vi "HaltDev.vi"(0 "输入簇":T1) -> ()   [LabVIEW 2012]
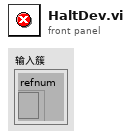
[diagram p1: front panel]
types:
  T1 = cluster{"refnum":refnum<file>, "refnum":refnum<file>, "refnum":refnum<file>, "refnum":refnum<file>, "refnum":refnum<file>, "SavePath":path, "SAVE?":bool, "connection ID":refnum<k5>}
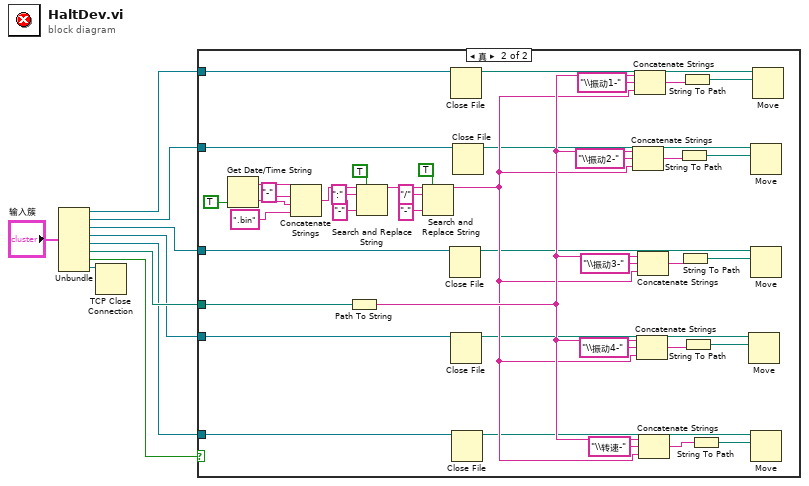
[diagram p0: block diagram]
diagram:
  n1 = Unbundle("输入簇") -> ("refnum"=w6:refnum<file>, "refnum"=w5:refnum<file>, "refnum"=w4:refnum<file>, "refnum"=w3:refnum<file>, "refnum"=w2:refnum<file>, "SavePath"=w7:path, "SAVE?"=w1:bool, "connection ID"=w8:refnum<k5>)
  n2 = TCP Close Connection(connection ID=w8) -> ()  [unwired: 2 in, 2 out]
  n3 = case shown="真" w1 {
    tunnel: w7 -> [_ w20]
    tunnel: w6 -> [_ w19]
    tunnel: w5 -> [_ w17]
    tunnel: w4 -> [_ w14]
    tunnel: w3 -> [_ w13]
    tunnel: w2 -> [_ w10]
    frame False {
    }
    frame True {
      n4 = Get Date/Time String(want seconds? (F)=TRUE ("需要秒？(F)")) -> (date string=w38:string, time string=w35:string)  [unwired: 2 in]
      n5 = Concatenate Strings(w38, "-" ("字符串"), w35, ".bin" ("字符串")) -> (w34:string)
      n6 = Path To String(path=w20) -> (string=w45:string)
      n7 = Search and Replace String(replace all?=TRUE ("替换全部？(F)"), input string=w34, search string=":" ("搜索字符串"), replace string="-" ("替换字符串(\"\")")) -> (result string=w27:string)  [unwired: 4 in, 3 out]
      n8 = Search and Replace String(replace all?=TRUE ("替换全部？(F)"), input string=w27, search string="/" ("搜索字符串"), replace string="-" ("替换字符串(\"\")")) -> (result string=w26:string)  [unwired: 4 in, 3 out]
      n9 = Close File(refnum=w14) -> (path=w15:path)  [unwired: 1 in, 1 out]
      n10 = Close File(refnum=w19) -> (path=w18:path)  [unwired: 1 in, 1 out]
      n11 = Close File(refnum=w13) -> (path=w12:path)  [unwired: 1 in, 1 out]
      n12 = Close File(refnum=w10) -> (path=w11:path)  [unwired: 1 in, 1 out]
      n13 = Close File(refnum=w17) -> (path=w16:path)  [unwired: 1 in, 1 out]
      n14 = Concatenate Strings(w45, "\\振动2-" ("字符串"), w26) -> (w47:string)
      n15 = Concatenate Strings(w45, "\\振动1-" ("字符串"), w26) -> (w46:string)
      n16 = Concatenate Strings(w45, "\\振动4-" ("字符串"), w26) -> (w49:string)
      n17 = Concatenate Strings(w45, "\\振动3-" ("字符串"), w26) -> (w48:string)
      n18 = Concatenate Strings(w45, "\\转速-" ("字符串"), w26) -> (w50:string)
      n19 = String To Path(string=w47) -> (path=w24:path)
      n20 = String To Path(string=w48) -> (path=w23:path)
      n21 = String To Path(string=w46) -> (path=w25:path)
      n22 = String To Path(string=w49) -> (path=w22:path)
      n23 = String To Path(string=w50) -> (path=w21:path)
      n24 = Move(source path=w12, 10:w22) -> ()  [unwired: 3 in, 3 out]
      n25 = Move(source path=w16, 10:w24) -> ()  [unwired: 3 in, 3 out]
      n26 = Move(source path=w15, 10:w23) -> ()  [unwired: 3 in, 3 out]
      n27 = Move(source path=w11, 10:w21) -> ()  [unwired: 3 in, 3 out]
      n28 = Move(source path=w18, 10:w25) -> ()  [unwired: 3 in, 3 out]
    }
  }
